vi "Check_Advise.vi"(0 "advise refnum":u32, 1 "Start Value":string, 2 "error in (no error)":errorcluster) -> (3 "advise refnum out":u32, 4 "current data":string, 5 "Value changed?":bool, 6 "error out":errorcluster)   [LabVIEW 2012]
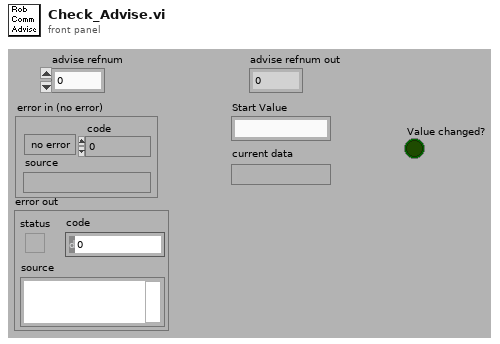
[diagram p1: front panel]
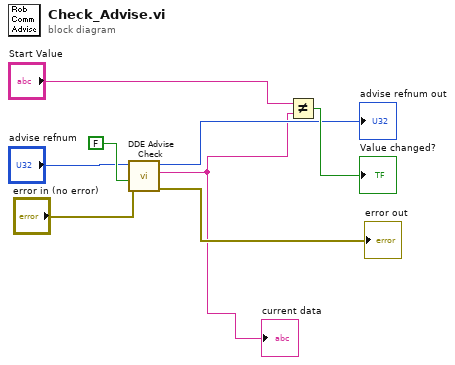
[diagram p0: block diagram]
diagram:
  n1 = call <vilib>:"DDE Advise Check.vi"("error in (no error)"="error in (no error)", "wait for change?(FALSE)"=FALSE, "advise refnum in"="advise refnum") -> ("error out"=→"error out":errorcluster, "current data"=w1:string, "advise refnum out"=→"advise refnum out":u32)  [unwired: 3 in, 1 out]
  "current data" <- w1
  n2 = Not Equal?(x="Start Value", y=w1) -> (x != y?=→"Value changed?":bool)
